vi "Get Basic VI Info.vi"() -> (2 "VI Description Info":T1)   [LabVIEW 2014]
uses:
  TYPE_Description Cluster.ctl
  TYPE_Version Status.ctl
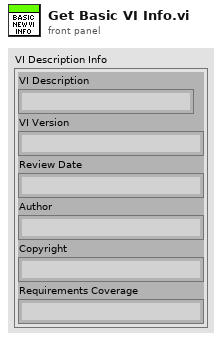
[diagram p1: front panel]
types:
  T1 = typedef "TYPE_Description Cluster.ctl" = cluster{"VI Description":string, "VI Version":string, "Review Date":string, "Author":string, "Copyright":string, "Requirements Coverage":string}
  T2 = typedef "TYPE_Version Status.ctl" = enum16{"Development", "alpha", "beta", "Reviewed", "Bug", "Other"}
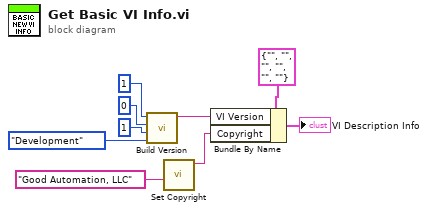
[diagram p0: block diagram]
diagram:
  n1 = call "Build Version.vi"("Current Phase"=TYPE_Version_Status."Development", "Revision"=u32 1, "Minor Revision"=u16 0, "Major Revision"=u16 1) -> ("VI Version"=w8:string)  [unwired: 7 in]
  n2 = call "Set Copyright.vi"("Company Name"="Good Automation, LLC") -> ("Updated Copyright"=w5:string)  [unwired: 10 in]
  n3 = Bundle By Name(cluster=T1 {"VI Description"="", "VI Version"="", "Review Date"="", "Author"="", "Copyright"="", "Requirements Coverage"=""} ("Description Cluster"), "VI Version"=w8, "Copyright"=w5) -> (→"VI Description Info":T1)
